vi "DAQ.vi"   [LabVIEW 2015]
uses:
  Controls/Channel Configuration.ctl
  CAN Communication/PAS/Typedefs/Session Handle.ctl
  CAN Communication/PAS/PAS.lvclass
  Common/Buffers/Snapshot/Typedefs/Session Handle.ctl
  Common/Buffers/Snapshot/Snapshot.lvclass
  Common/Circular Error Log/Typedefs/Session Handle.ctl
  Common/Circular Error Log/Circular Error Log.lvclass
  Config/User Configuration.ctl
  Common/State Machine/State Machine.lvlib
  User Interface/UI Handler/UI Handler.lvclass
panel:
  # "DAQ"
types:
  T1 = typedef "Channel Configuration.ctl" = cluster{"Index":u16, "Name":string, "Units":string, "Gain":dbl, "Offset":dbl, "Source":string}
  T2 = typedef "PAS.lvclass/Session Handle.ctl" = refnum<data-value>
  T3 = typedef "Snapshot.lvclass/Session Handle.ctl" = refnum<data-value>
  T4 = typedef "Circular Error Log.lvclass/Session Handle.ctl" = refnum<data-value>
  T5 = typedef "User Configuration.ctl" = cluster{"Password":string, "cDAQ Name":string, "CAN Interface":string}
  T6 = cluster{"State":refnum<queue>, "Channels":T1[], "PAS":T2, "Snapshot":T3, "LogData":refnum<queue>, "Error":T4, "Alerted?":bool, "User Config":T5}
  T7 = cluster{"Averaged Values":dbl[], "seconds since 1Jan1904":timestamp}
  T8 = cluster{"Values":dbl[], "seconds since 1Jan1904":timestamp}
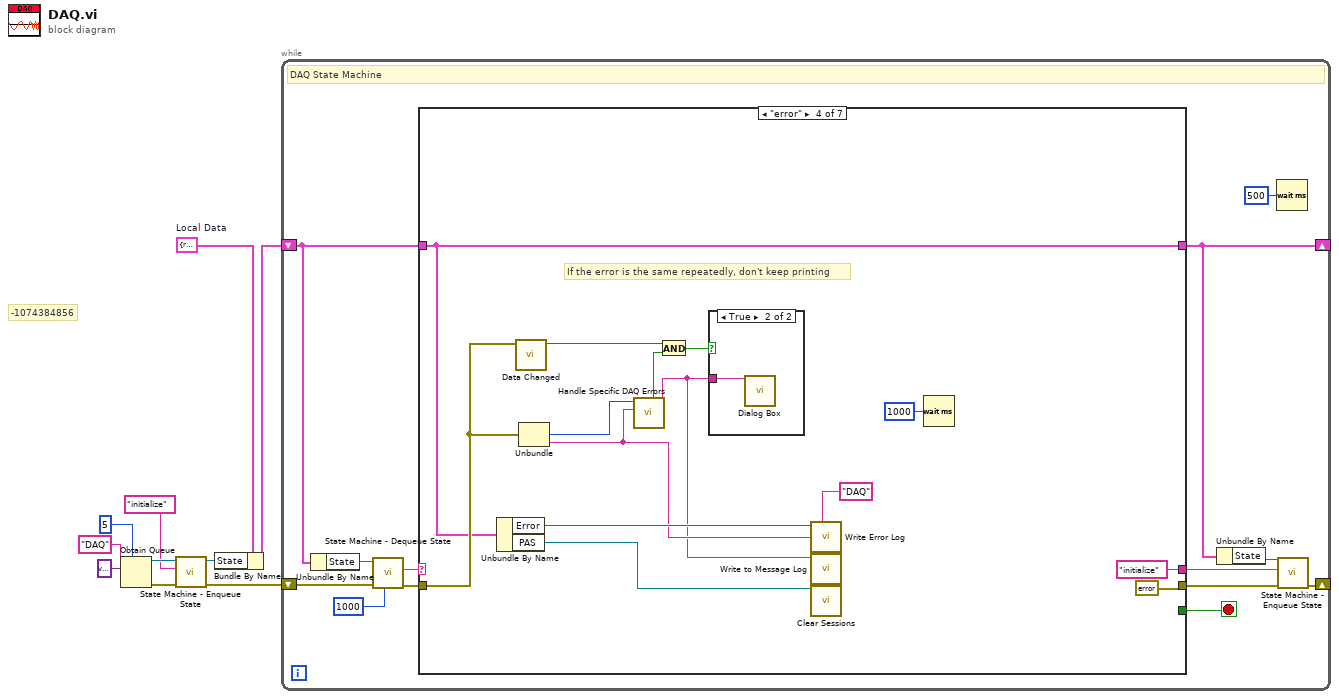
[diagram p0: block diagram]
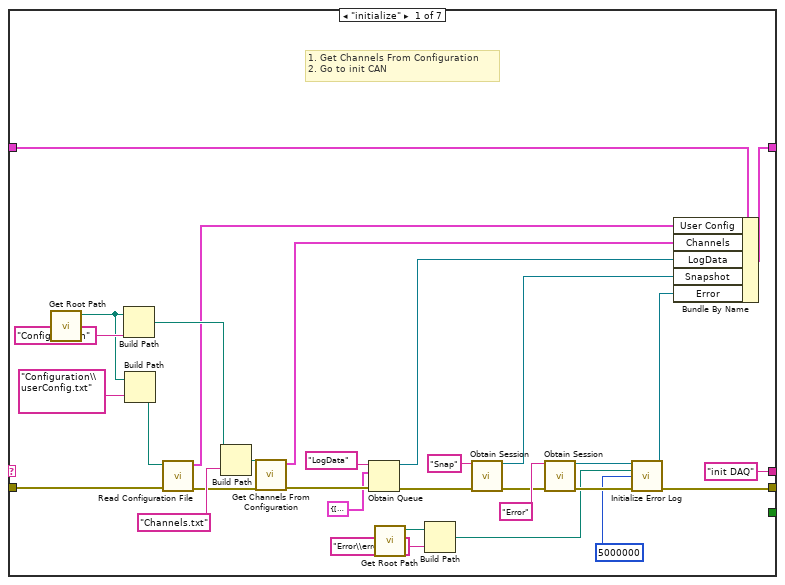
[diagram p2: hidden frame]
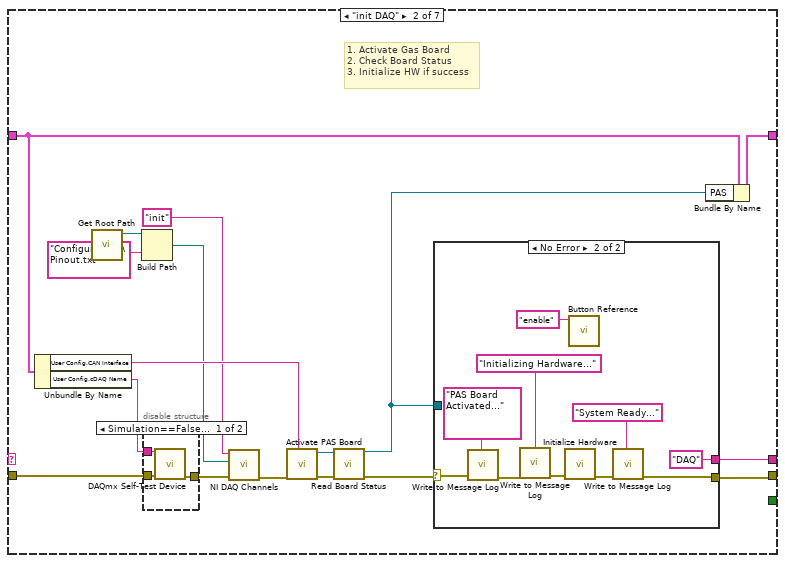
[diagram p3: hidden frame]
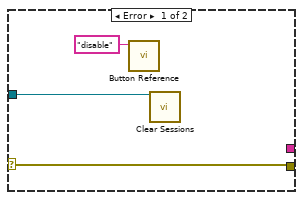
[diagram p5: hidden frame]
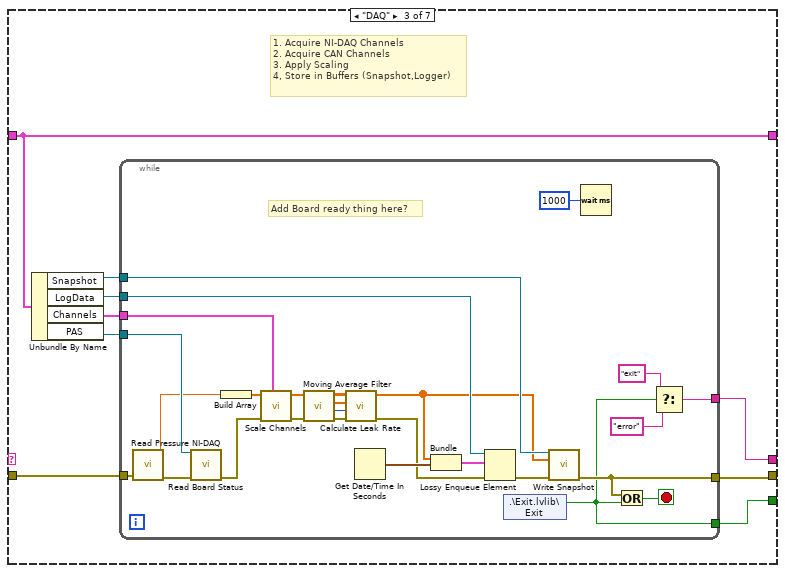
[diagram p6: hidden frame]
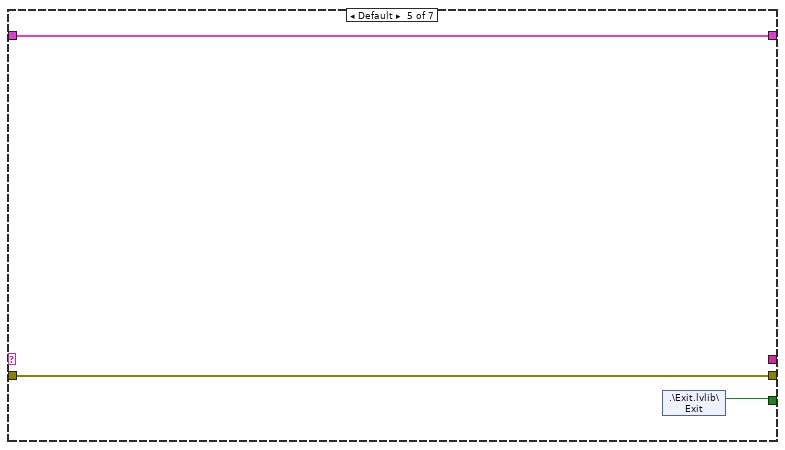
[diagram p8: hidden frame]
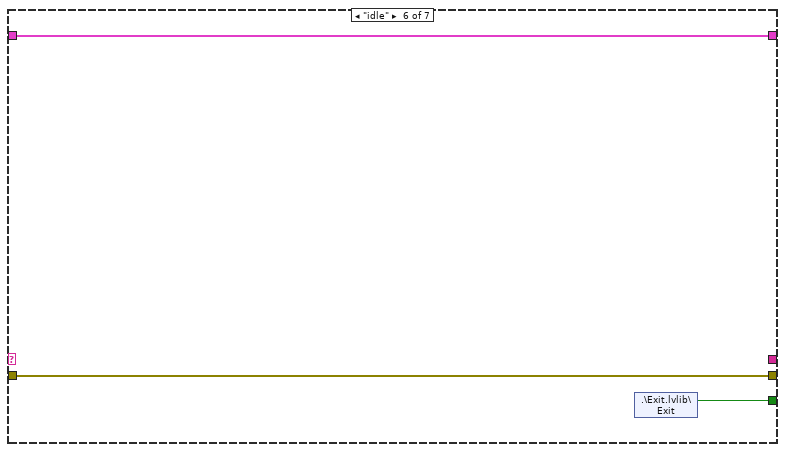
[diagram p9: hidden frame]
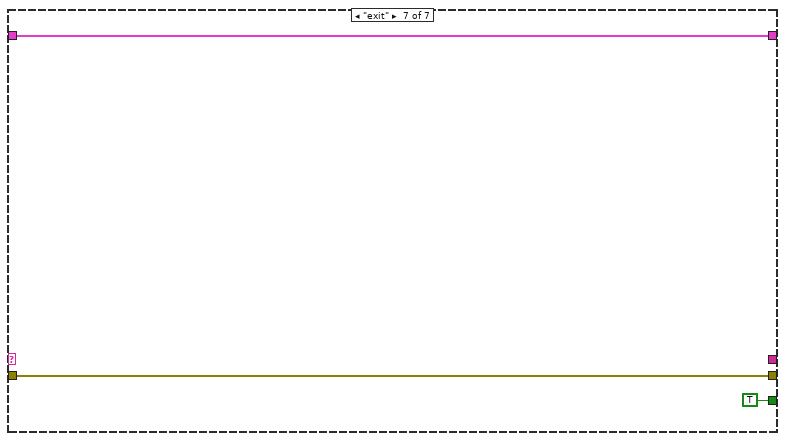
[diagram p10: hidden frame]
diagram:
  w3 = T6 {"State"=refnum, "Channels"=[], "PAS"=refnum, "Snapshot"=refnum, "LogData"=refnum, "Error"=refnum, "Alerted?"=FALSE, "User Config"={"Password"="", "cDAQ Name"="", "CAN Interface"=""}}  # Local Data
  # "-1074384856"
  n1 = Obtain Queue(max queue size (-1, unlimited)=5, name (unnamed)="DAQ", element data type=variant) -> (queue out=w6:refnum<queue>, error out=w7:errorcluster)  [unwired: 2 in, 1 out]
  n2 = call "State Machine - Enqueue State.vi"("error in (no error)"=w7, "State"="initialize", "Queue In"=w6) -> ("error out"=w4:errorcluster, "Queue Out"=w2:refnum<queue>)  [unwired: 7 in]
  n3 = Bundle By Name(cluster=w3, "State"=w2) -> (w1:T6)
  n4 = while "Main State Machine" {
    shift-right: [w20] -> _
    shift-left: w4 -> [w23]
    shift-right: [w11] -> _
    shift-left: w1 -> [w14]
    stop <- w16 stop-if-true
    # "DAQ State Machine"
    n5 = Unbundle By Name(w14) -> ("State"=w13:refnum<queue>)
    n6 = call "State Machine - Dequeue State.vi"("Timeout"=1000, "error in (no error)"=w23, "Queue In"=w13) -> ("error out"=w22:errorcluster, "State"=w21:string)  [unwired: 4 in, 3 out]
    n7 = case shown="\"error\"" w21 {
      tunnel: w22 -> [w29 w67 w97 w135 w142 w145 w148]
      tunnel: [w33 w70 w94 errorcluster {"status"=FALSE, "code"=0, "source"=""} ("error out") w142 w145 w148] -> w19
      tunnel: ["init DAQ" ("State") w69 w91 "initialize" ("State") _ _ _] -> w18
      tunnel: [_ _ w90 _ w140 w143 TRUE] -> w16
      tunnel: w14 -> [w50 w68 w96 w134 w141 w144 w146]
      tunnel: [w49 w71 w96 w134 w141 w144 w146] -> w11
      frame "initialize" {
        # "1. Get Channels From Configuration\n2. Go to init CAN"
        n8 = call "Get Root Path.vi"() -> ("Root Path"=w26:path)  [unwired: 11 in]
        n9 = Build Path(base path=w26, name or relative path="Configuration") -> (appended path=w53:path)
        n10 = Build Path(base path=w26, name or relative path="Configuration\\userConfig.txt") -> (appended path=w24:path)
        n11 = call "Read Configuration File.vi"("error in (no error)"=w29, "Filepath"=w24) -> ("error out"=w28:errorcluster, "User Config"=w27:T5)  [unwired: 8 in]
        n12 = Build Path(base path=w53, name or relative path="Channels.txt") -> (appended path=w51:path)
        n13 = call "Get Channels From Configuration.vi"("error in (no error)"=w28, "Path"=w51) -> ("error out"=w47:errorcluster, "Channels"=w48:T1[])  [unwired: 8 in]
        n14 = Obtain Queue(name (unnamed)="LogData", element data type=T7 {"Averaged Values"=[], "seconds since 1Jan1904"=timestamp(0 s since 1904-01-01)} ("output cluster"), error in (no error)=w47) -> (queue out=w41:refnum<queue>, error out=w45:errorcluster)  [unwired: 2 in, 1 out]
        n15 = call "Get Root Path.vi"() -> ("Root Path"=w32:path)  [unwired: 11 in]
        n16 = Build Path(base path=w32, name or relative path="Error\\error.txt") -> (appended path=w30:path)
        n17 = call "Obtain Session.vi"("Session  Name ()"="Snap", "error in (no error)"=w45) -> ("Session Handle"=w43:T3, "error out"=w35:errorcluster)  [unwired: 12 in]
        n18 = call "Obtain Session.vi"("Session  Name ()"="Error", "error in (no error)"=w35) -> ("Session Handle"=w37:T4, "error out"=w38:errorcluster)  [unwired: 12 in]
        n19 = call "Initialize Error Log.vi"("Session Handle in"=w37, "Error Path"=w30, "Max File Size"=i64 5000000, "error in (no error)"=w38) -> ("Session Handle out"=w34:T4, "error out"=w33:errorcluster)  [unwired: 10 in]
        n20 = Bundle By Name(cluster=w50, "User Config"=w27, "Channels"=w48, "LogData"=w41, "Snapshot"=w43, "Error"=w34) -> (w49:T6)
      }
      frame "init DAQ" {
        # "1. Activate Gas Board\n2. Check Board Status\n3. Initialize HW if success"
        n21 = Unbundle By Name(w68) -> ("User Config.CAN Interface"=w61:string, "User Config.cDAQ Name"=w66:string)
        n22 = call "Get Root Path.vi"() -> ("Root Path"=w59:path)  [unwired: 11 in]
        n23 = Build Path(base path=w59, name or relative path="Configuration\\Pinout.txt") -> (appended path=w55:path)
        n24 = disable-structure shown="Simulation==False, Default" {
          disable-tunnel: w67 -> [w74 w75]
          disable-tunnel: [w73 w75] -> w58
          disable-tunnel: w66 -> [w72 _]
          frame condition #0 (active) {
            n25 = call <vilib>:"DAQmx Self-Test Device.vi"("device in"=w72, "error in"=w74) -> ("error out"=w73:errorcluster)  [unwired: 13 in]
          }
          frame condition #1 {
          }
        }
        n26 = call "NI DAQ Channels.vi"("error in (no error)"=w58, "Path"=w55, "Command"="init" ("name or relative path")) -> ("error out"=w57:errorcluster)  [unwired: 7 in, 1 out]
        n27 = call "Activate PAS Board.vi"("CAN Interface"=w61, "error in (no error)"=w57) -> ("error out"=w65:errorcluster, "Session Handle out"=w64:T2)  [unwired: 8 in]
        n28 = call "Read Board Status.vi"("Session Handle in"=w64, "error in (no error)"=w65) -> ("Session Handle out"=w63:T2, "error out"=w62:errorcluster)  [unwired: 11 in, 1 out]
        n29 = case shown="No Error" w62 {
          selector: w62 -> [w77 w86]
          tunnel: [w77 w81] -> w70
          tunnel: [_ "DAQ" ("State")] -> w69
          tunnel: w63 -> [w78 _]
          frame Error {
            n30 = call "Button Reference.vi"("Command"="disable") -> ()  [unwired: 10 in, 1 out]
            n31 = call "Clear Sessions.vi"("Session Handle in"=w78) -> ()  [unwired: 13 in, 2 out]
          }
          frame No Error {
            n32 = call "Write to Message Log.vi"("error in (no error)"=w86, "Message"="PAS Board Activated...") -> ("error out"=w82:errorcluster)  [unwired: 9 in]
            n33 = call "Write to Message Log.vi"("error in (no error)"=w82, "Message"="Initializing Hardware...") -> ("error out"=w85:errorcluster)  [unwired: 9 in]
            n34 = call "Initialize Hardware.vi"("error in"=w85) -> ("error out"=w83:errorcluster)  [unwired: 10 in]
            n35 = call "Button Reference.vi"("Command"="enable") -> ()  [unwired: 10 in, 1 out]
            n36 = call "Write to Message Log.vi"("error in (no error)"=w83, "Message"="System Ready...") -> ("error out"=w81:errorcluster)  [unwired: 9 in]
          }
        }
        n37 = Bundle By Name(cluster=w68, "PAS"=w63) -> (w71:T6)
      }
      frame "DAQ" {
        # "1. Acquire NI-DAQ Channels\n2. Acquire CAN Channels \n3. Apply Scaling\n4, Store in Buffers (Snapshot,Logger)"
        n38 = Unbundle By Name(w96) -> ("Snapshot"=w92:T3, "LogData"=w93:refnum<queue>, "Channels"=w95:T1[], "PAS"=w89:T2)
        n39 = while {
          tunnel: w97 -> [w109]
          tunnel: w89 -> [w101]
          tunnel: w95 -> [w124]
          tunnel: [w117] -> w94
          tunnel: w93 -> [w120]
          tunnel: w92 -> [w118]
          tunnel: [w113] -> w91
          tunnel: [w112] -> w90
          stop <- w121 stop-if-true
          # "Add Board ready thing here?"
          n40 = call "Read Pressure NI-DAQ.vi"("error in (no error)"=w109) -> ("error out"=w102:errorcluster, "Pressure"=w99:dbl)  [unwired: 9 in]
          n41 = call "Read Board Status.vi"("Session Handle in"=w101, "error in (no error)"=w102) -> ("error out"=w100:errorcluster)  [unwired: 11 in, 2 out]
          n42 = Build Array(w99) -> (w108:dbl[])
          n43 = call "Scale Channels.vi"("Config"=w124, "error in (no error)"=w100, "Channels In"=w108) -> ("error out"=w123:errorcluster, "Channels Out"=w122:dbl[])  [unwired: 7 in]
          n44 = call "Moving Average Filter.vi"("error in (no error)"=w123, "Values"=w122) -> ("error out"=w104:errorcluster, "Count"=w105:i32, "Averaged Values"=w106:dbl[], "Buffer"=w107:dbl[][])  [unwired: 6 in]
          n45 = call "Calculate Leak Rate.vi"("error in (no error)"=w104, "Count"=w105, "Averaged Values"=w106, "Buffer"=w107) -> ("error out"=w103:errorcluster, "Values"=w98:dbl[])  [unwired: 6 in]
          n46 = Get Date/Time In Seconds() -> (seconds since 1Jan1904=w111:timestamp)
          n47 = Bundle("Values"=w98, "seconds since 1Jan1904"=w111) -> (w110:T8)  [unwired: 1 in]
          n48 = Lossy Enqueue Element(queue=w120, element=w110, error in (no error)=w103) -> (error out=w119:errorcluster)  [unwired: 3 out]
          n49 = shared-variable ".\\Exit.lvlib\\Exit"() -> (w112:bool)  [unwired: 1 in, 1 out]
          n50 = call "Write Snapshot.vi"("Session Handle in"=w118, "Buffer"=w98, "error in (no error)"=w119) -> ("error out"=w117:errorcluster)  [unwired: 11 in, 1 out]
          n51 = Wait (ms)(milliseconds to wait=u32 1000) -> ()  [unwired: 1 out]
          n52 = Or(x=w117, y=w112) -> (x .or. y?=w121:bool)
          n53 = Select(t="exit" ("State"), s=w112, f="error" ("State")) -> (s? t:f=w113:string)
        }
      }
      frame "error" {
        # "If the error is the same repeatedly, don't keep printing"
        n54 = Unbundle By Name(w134) -> ("Error"=w136:T4, "PAS"=w126:T2)
        n55 = call "Data Changed.vi"("Data"=w135) -> ("Changed?"=w128:bool)  [unwired: 10 in]
        n56 = Unbundle(w135) -> ("code"=w133:i32, "source"=w130:string)  [unwired: 1 out]
        n57 = call "Handle Specific DAQ Errors.vi"("Error In"=w130, "code"=w133) -> ("Error Message"=w125:string, "Alert User?"=w127:bool)  [unwired: 7 in, 1 out]
        n58 = And(x=w128, y=w127) -> (x .and. y?=w129:bool)
        n59 = case shown="True" w129 {
          tunnel: w125 -> [_ w139]
          frame False {
          }
          frame True {
            n60 = call "Dialog Box.vi"("Serial Number"=w139) -> ()  [unwired: 10 in, 1 out]
          }
        }
        n61 = call "Write Error Log.vi"("Session Handle in"=w136, "Process Name"="DAQ", "Data"=w130) -> ()  [unwired: 11 in, 2 out]
        n62 = call "Write to Message Log.vi"("Message"=w125) -> ()  [unwired: 10 in, 1 out]
        n63 = call "Clear Sessions.vi"("Session Handle in"=w126) -> ()  [unwired: 13 in, 2 out]
        n64 = Wait (ms)(milliseconds to wait=u32 1000) -> ()  [unwired: 1 out]
      }
      frame Default {
        n65 = shared-variable ".\\Exit.lvlib\\Exit"() -> (w140:bool)  [unwired: 1 in, 1 out]
      }
      frame "idle" {
        n66 = shared-variable ".\\Exit.lvlib\\Exit"() -> (w143:bool)  [unwired: 1 in, 1 out]
      }
      frame "exit" {
      }
    }
    n67 = Unbundle By Name(w11) -> ("State"=w12:refnum<queue>)
    n68 = Wait (ms)(milliseconds to wait=u32 500) -> ()  [unwired: 1 out]
    n69 = call "State Machine - Enqueue State.vi"("error in (no error)"=w19, "State"=w18, "Queue In"=w12) -> ("error out"=w20:errorcluster)  [unwired: 7 in, 1 out]
  }
